vi "StreamingTest.vi"() -> ()   [LabVIEW 2016]
uses:
  <vilib>/Instr/_visa.llb/VISA Configure Serial Port (Instr).vi
panel:
  out "#error":i32
  out "Freq":dbl
  out "Time":dbl[](array[numeric])
  out "Reading":string[](array[string])
  in  "VISA resource name":refnum<visa-resource-name>="COM4"
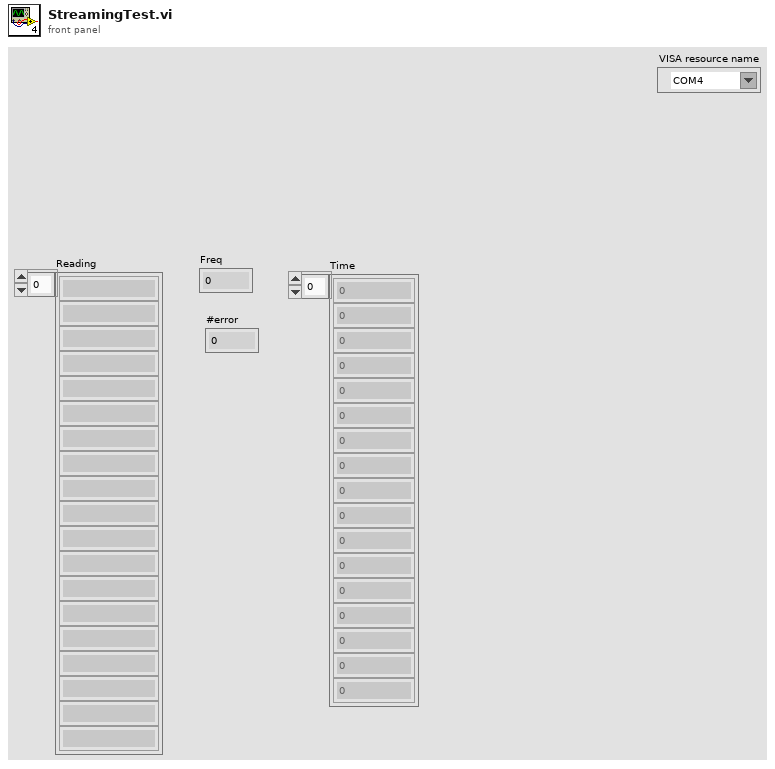
[diagram p1: front panel]
types:
  T1 = enum16{"SetLock", "UnSetLock", "Read", "SetStreamMode", "UnSetStreammingMode"}
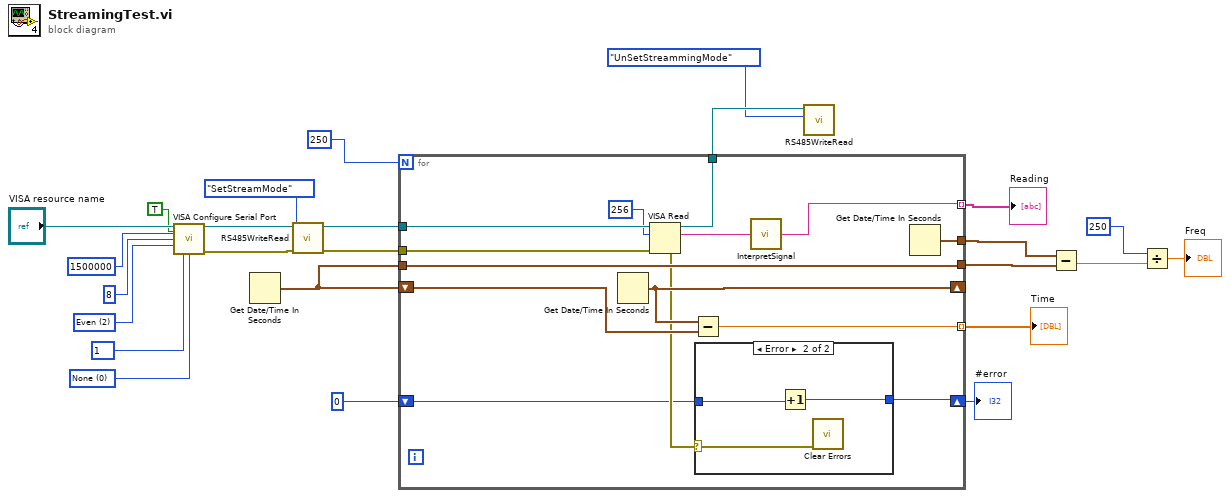
[diagram p0: block diagram]
diagram:
  w23 = u16 0 items=["None"=0, "XON/XOFF"=1, "RTS/CTS"=2, "DTR/DSR"=4] ("flow control")
  w22 = u16 10 items=["1"=10, "1.5"=15, "2.0"=20] ("stop bits")
  w21 = u16 2 items=["None", "Odd", "Even", "Mark", "Space"] ("parity")
  n1 = call-poly "VISA Configure Serial Port"("VISA resource name"="VISA resource name", "Enable Termination\nChar (T)"=TRUE, "baud rate (9600)"=u32 1500000 ("baud rate"), "data bits (8)"=u16 8 ("data bits"), "parity (0:none)"=w21, "stop bits (10: 1 bit)"=w22, "flow control (0:none)"=w23) -> ("VISA resource name out"=w2:refnum<visa-resource-name>, "error out"=w3:errorcluster)  [unwired: 7 in]
  n2 = Get Date/Time In Seconds() -> (seconds since 1Jan1904=w17:timestamp)
  n3 = call "RS485WriteRead.vi"("error in (no error)"=w3, "Control Option"=T1."SetStreamMode", "VISA resource name"=w2) -> ("error out"=w4:errorcluster, "VISA resource name out"=w5:refnum<visa-resource-name>)  [unwired: 6 in, 1 out]
  n4 = for {
    N: 250 -> [_]
    tunnel: w5 -> [w39]
    tunnel: w4 -> [w38]
    shift-right: [w36] -> _
    shift-left: w17 -> [w37]
    tunnel: w17 -> [w34]
    tunnel: [w34] -> w16
    tunnel: [w33] -> w7
    tunnel: [w32] -> w15 mode=indexing
    tunnel: [w30] -> w14
    tunnel: [w28] -> w10 mode=indexing
    shift-right: [w26] -> w8
    shift-left: 0 -> [w27]
    n5 = Get Date/Time In Seconds() -> (seconds since 1Jan1904=w36:timestamp)
    n6 = VISA Read(VISA resource name=w39, byte count=256, error in (no error)=w38) -> (VISA resource name out=w33:refnum<visa-resource-name>, read buffer=w35:string, error out=w29:errorcluster)  [unwired: 1 out]
    n7 = Subtract(x=w36, y=w37) -> (x-y=w32:dbl)
    n8 = case shown="Error" w29 {
      selector: w29 -> [_ w43]
      tunnel: w27 -> [w40 w42]
      tunnel: [w40 w41] -> w26
      frame No Error {
      }
      frame Error {
        n9 = Increment(x=w42) -> (x+1=w41:i32)
        n10 = call <vilib>:"Clear Errors.vi"("error in (no error)"=w43) -> ()  [unwired: 5 in, 2 out]
      }
    }
    n11 = call "InterpretSignal.vi"("String in"=w35) -> ("String out"=w28:string)
    n12 = Get Date/Time In Seconds() -> (seconds since 1Jan1904=w30:timestamp)
  }
  "Reading" <- w10
  "Time" <- w15
  "#error" <- w8
  n13 = call "RS485WriteRead.vi"("Control Option"=T1."UnSetStreammingMode", "VISA resource name"=w7) -> ()  [unwired: 7 in, 3 out]
  n14 = Subtract(x=w14, y=w16) -> (x-y=w12:dbl)
  n15 = Divide(x=250, y=w12) -> (x/y=→"Freq":dbl)
